vi "Get Target IP Address.vi"(8 "error in (no error)":errorcluster, 11 "Item Ref in":T1 format="%.0x") -> (0 "error out":errorcluster, 1 "found":bool, 2 "target address":string, 3 "Item Ref out":T1 format="%.0x")   [LabVIEW 2020, in "DSF System Explorer.lvlib"]
uses:
  DSF System Explorer.lvlib
  <vilib>/NI VeriStand/Custom Device API/Custom Device Item Ref.ctl
  NationalInstruments.VeriStand.SystemDefinitionAPI
  NationalInstruments.VeriStand.SystemStorage
  <vilib>/NI VeriStand/Custom Device API/Custom Device API.lvlib
  <vilib>/NI VeriStand/Custom Device Offline API/Custom Device Offline API.lvlib
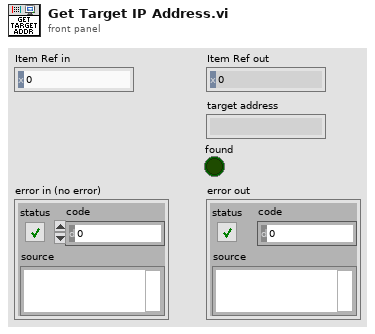
[diagram p1: front panel]
types:
  T1 = typedef "Custom Device API.lvlib/Custom Device Item Ref.ctl" = u64
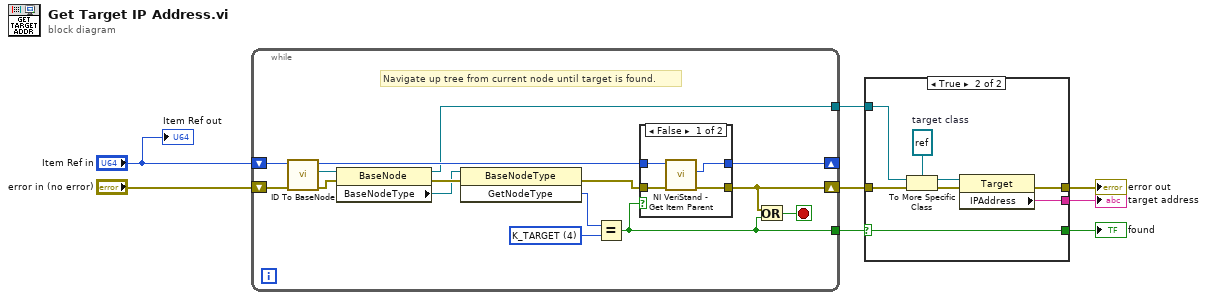
[diagram p0: block diagram]
diagram:
  n1 = while {
    shift-right: [w20] -> _
    shift-left: "Item Ref in" -> [w13]
    shift-right: [w11] -> w8
    shift-left: "error in (no error)" -> [w18]
    tunnel: [w10] -> w5
    tunnel: [w12] -> w1
    stop <- w9 stop-if-true
    w21 = 4 items=["K_BASE", "K_ALIAS", "K_CHANNEL", "K_SECTION", "K_TARGET", "K_TARGETSECTION", "K_ROOT", "K_WAVEFORM", "K_PARAMETER"] ("GetNodeType")
    # "Navigate up tree from current node until target is found."
    n2 = call <vilib>:"ID To BaseNode.vi"("error in (no error)"=w18, "ID in"=w13) -> ("error out"=w17:errorcluster, "BaseNode"=w16:refnum<k24>)  [unwired: 7 in, 1 out]
    n3 = property class="BaseNode"(reference=w16, error in=w17) -> (reference out=w12:refnum<k24>, error out=w15:errorcluster, "BaseNodeType"=w14:refnum<k24>)
    n4 = invoke class="BaseNodeType" method="GetNodeType"(reference=w14, error in=w15) -> (error out=w19:errorcluster, "GetNodeType"=w22:i32)  [unwired: 1 in, 1 out]
    n5 = Equal?(x=w22, y=w21) -> (x = y?=w10:bool)
    n6 = case shown="False" w10 {
      tunnel: [w26 w28] -> w11
      tunnel: w19 -> [w25 w28]
      tunnel: [w24 w27] -> w20
      tunnel: w13 -> [w23 w27]
      frame False {
        n7 = call <vilib>:"NI VeriStand - Get Item Parent.vi"("error in (no error)"=w25, "Item Ref in"=w23) -> ("error out"=w26:errorcluster, "Parent Ref"=w24:T1)  [unwired: 6 in, 2 out]
      }
      frame True {
      }
    }
    n8 = Or(x=w11, y=w10) -> (x .or. y?=w9:bool)
  }
  n9 = case shown="True" w5 {
    selector: w5 -> [w29 w31]
    tunnel: w8 -> [w30 w35]
    tunnel: [w30 w38] -> w7
    tunnel: [_ w37] -> w6
    tunnel: [w29 w31] -> w4
    tunnel: w1 -> [_ w36]
    frame False {
    }
    frame True {
      w32 = refnum<k24> refnum  # target class
      n10 = To More Specific Class(target class=w32, reference=w36, error in=w35) -> (specific class reference=w34:refnum<k24>, error out=w33:errorcluster)
      n11 = property class="Target"(reference=w34, error in=w33) -> (error out=w38:errorcluster, "IPAddress"=w37:string)  [unwired: 1 out]
    }
  }
  "error out" <- w7
  "target address" <- w6
  "found" <- w4
  "Item Ref out" <- "Item Ref in"
